vi "Init Splash.vi"(8 "error in (no error)":errorcluster, 11 "Plugin Splash in":refnum<class "Plugin Splash.lvclass">) -> (0 "error out":errorcluster, 3 "Plugin Splash out":refnum<class "Plugin Splash.lvclass">)   [LabVIEW 2020, in "Volatus.lvlib" / "Plugin Splash.lvclass"]
uses:
  Plugin Splash.lvclass
  Plugin Splash.lvclass/Plugin Splash.ctl
  splash.vi
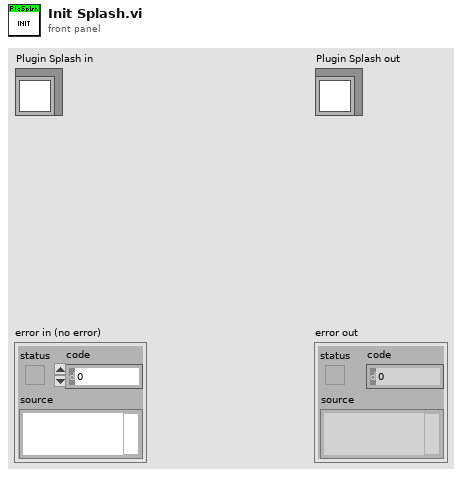
[diagram p1: front panel]
types:
  T1 = enum32{"Invalid", "Standard", "Closed", "Hidden", "Minimized", "Maximized"}
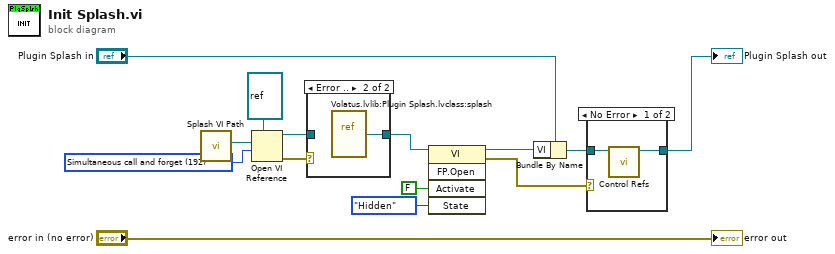
[diagram p0: block diagram]
diagram:
  w12 = 192 items=["Record modifications"=1, "Open templates for editing"=2, "Prompt user to save"=4, "Prepare for reentrant run"=8, "Prompt to find missing subVIs"=16, "Hide loading dialog box"=32, "Enable simultaneous calls"=64, "Prepare to call and forget"=128, "Simultaneous call and forget"=192, "Prepare to call and collect"=256, "Simultaneous call and collect"=320]
  n1 = call "Splash VI Path.vi"() -> ("Splash VI Path"=w9:path)  [unwired: 11 in]
  n2 = Open VI Reference(type specifier VI Refnum (for type only)=refnum<vi> refnum, vi path=w9, options=w12) -> (vi reference=w2:refnum<vi>, error out=w3:errorcluster)  [unwired: 3 in]
  n3 = case shown="Error .." w3 {
    tunnel: w2 -> [w15 _]
    tunnel: [w15 w16] -> w1
    frame No Error {
    }
    frame Error {
      n4 = vi-ref "Volatus.lvlib:Plugin Splash.lvclass:splash.vi"() -> (w16:refnum<vi>)
    }
  }
  n5 = invoke class="VI" method="FP.Open"(reference=w1, "Activate"=FALSE ("Activate?"), "State"=T1."Hidden") -> (reference out=w6:refnum<vi>, error out=w4:errorcluster)  [unwired: 2 in, 3 out]
  n6 = Bundle By Name(cluster="Plugin Splash in", "VI"=w6) -> (w7:refnum<class "Plugin Splash.lvclass">)
  n7 = case shown="No Error" w4 {
    tunnel: w7 -> [w18 w19]
    tunnel: [w17 w19] -> w5
    frame No Error {
      n8 = call "Control Refs.vi"("Plugin Splash in"=w18) -> ("Plugin Splash out"=w17:refnum<class "Plugin Splash.lvclass">)  [unwired: 9 in, 1 out]
    }
    frame Error {
    }
  }
  "Plugin Splash out" <- w5
  "error out" <- "error in (no error)"
